vi "LoadZstackImages.vi"(0 "Experiment folder path OR Z-stack folder path":path, 11 "Error In":errorcluster) -> (1 "Number of Files":i32, 2 "All outputs":T2, 3 "AOL Z Planes":dbl[](array[numeric]), 4 "RedImageArray":T1[](array[typedef]), 6 "GreenImageArray":T1[](array[typedef]), 8 "Motor Z planes":dbl[](array[numeric]), 10 "AOL Z Planes (norm)":dbl[](array[numeric]), 12 "RedMaxZ":T1, 14 "GreenMaxZ":T1, 15 "Error Out":errorcluster)   [LabVIEW 2013]
uses:
  <vilib>/vision/Image Controls.llb/IMAQ Image.ctl
  <vilib>/vision/NI_Vision_Development_Module.lvlib
panel:
  out "Green":path[](array[path])
  out "Red":path[](array[path])
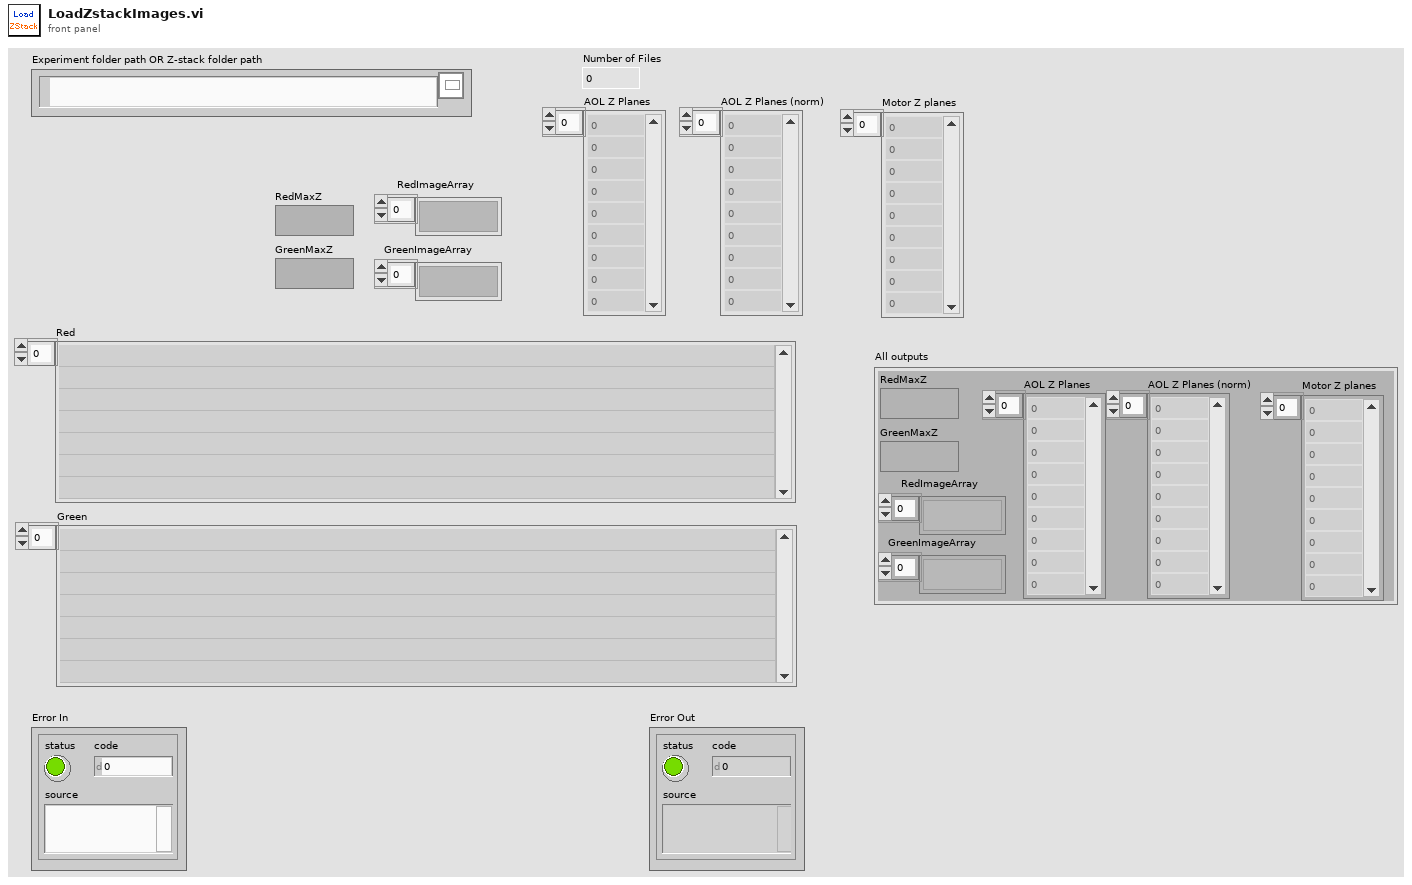
[diagram p1: front panel]
types:
  T1 = typedef "IMAQ Image.ctl" = refnum<image>
  T2 = cluster{"RedImageArray":T1[], "GreenImageArray":T1[], "RedMaxZ":T1, "GreenMaxZ":T1, "AOL Z Planes":dbl[], "AOL Z Planes (norm)":dbl[], "Motor Z planes":dbl[]}
  T3 = typedef "Fixed strings.ctl" = cluster{"ROI file name":string, "Normalised ROI file name":string, "Zplane Pockels values file name":string, "Functional data folder name":string, "Experiment Header file name":string, "Z-stack images folder name":string, "Groups setup rel. path":string, "Groups text file rel. path":string, "TDMS files folder name (F.img)":string, "TDMS files folder name (V.acq)":string, "TDMS files folder name (Pl.acq)":string, "Cycle rel times sequence file":string, "Dynamically called VIs folder name":string, "Time Series folder base name":string}
  T4 = enum32{"Average", "Min", "Max", "Clear  if < ", "Clear  if < or =", "Clear  if =", "Clear  if > or =", "Clear  if >"}
  T5 = typedef "Image Type" = u32
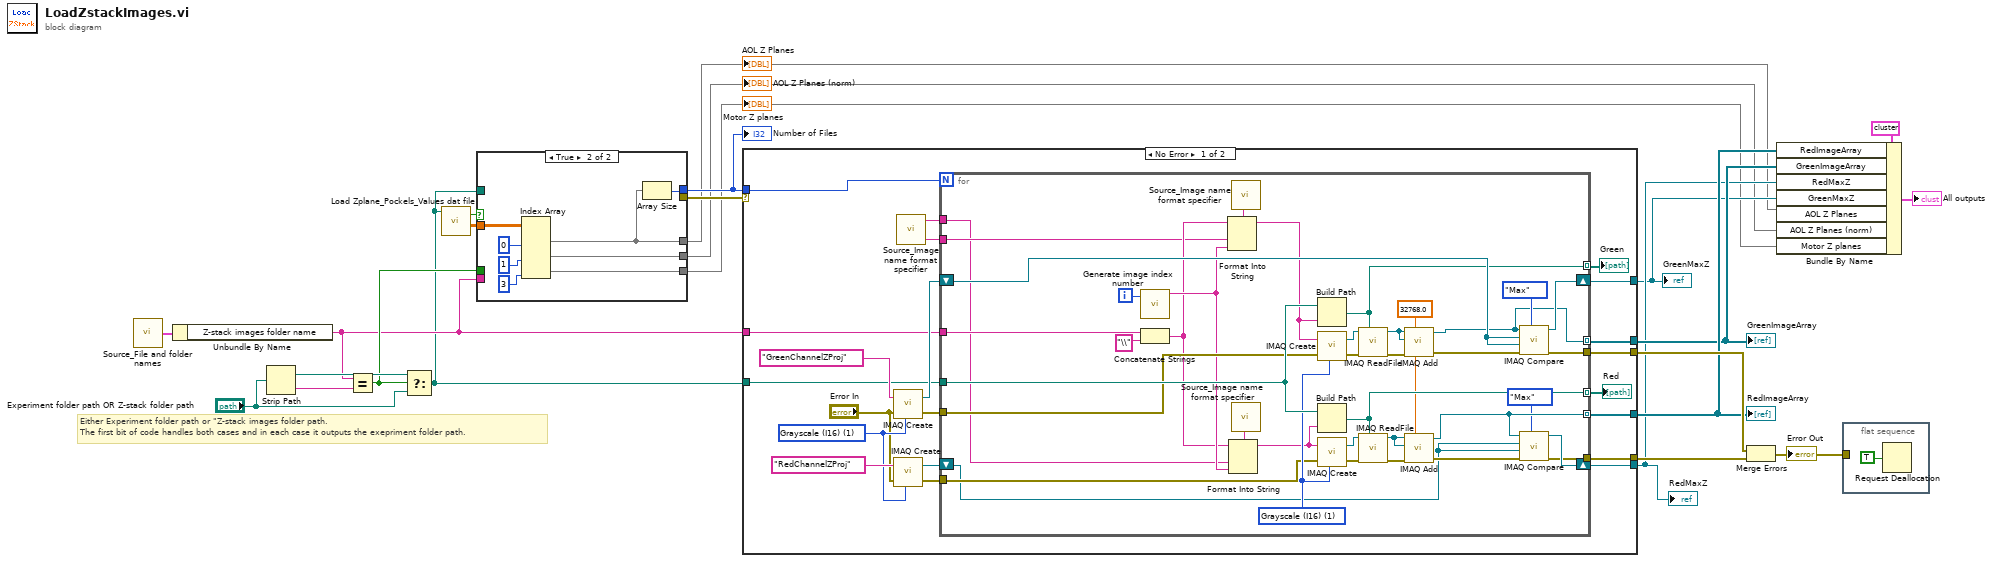
[diagram p0: block diagram]
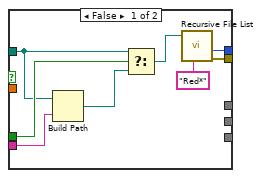
[diagram p2: hidden frame]
diagram:
  # "Either Experiment folder path or \"Z-stack images folder path.\nThe first bit of code handles both cases and in each case it outputs the exepriment folder path."
  n1 = call "Source_File and folder names.vi"() -> ("Fixed strings"=w15:T3)  [unwired: 1 in]
  n2 = Unbundle By Name(w15) -> ("Z-stack images folder name"=w14:string)
  n3 = Strip Path(path="Experiment folder path OR Z-stack folder path") -> (stripped path=w21:path, name=w18:string)
  n4 = Equal?(x=w14, y=w18) -> (x = y?=w20:bool)
  n5 = Select(t=w21, s=w20, f="Experiment folder path OR Z-stack folder path") -> (s? t:f=w1:path)
  n6 = call "Load Zplane_Pockels_Values dat file.vi"("Experiment data folder path"=w1) -> ("Zplane_Pockels_Values file data (header removed)"=w13:dbl[][], "Zplane Pockels values file exists"=w12:bool)  [unwired: 5 in, 4 out]
  n7 = case shown="True" w12 {
    tunnel: [w30 w38] -> w16
    tunnel: w1 -> [w27 _]
    tunnel: w14 -> [w29 _]
    tunnel: w20 -> [w28 _]
    tunnel: [w24 _] -> w19
    tunnel: [_ w36] -> w4
    tunnel: [_ w35] -> w3
    tunnel: w13 -> [_ w34]
    tunnel: [_ w32] -> w2
    frame False {
      n8 = Build Path(base path=w27, name or relative path=w29) -> (appended path=w26:path)
      n9 = Select(t=w27, s=w28, f=w26) -> (s? t:f=w25:path)
      n10 = call <vilib>:"Recursive File List.vi"("pattern"="Red*", "Folder Path"=w25) -> ("error out"=w24:errorcluster, "Number of Files"=w30:i32)  [unwired: 5 in, 3 out]
    }
    frame True {
      n11 = Index Array(array=w34, index (col) #1=0 ("disabled index (col)"), index (col) #2=1 ("disabled index (row)"), index (col) #3=3 ("index (col)")) -> (element #1=w36:dbl[], element #2=w35:dbl[], element #3=w32:dbl[])  [unwired: 3 in]
      n12 = Array Size(array=w36) -> (size(s)=w38:i32)
    }
  }
  "AOL Z Planes" <- w4
  "AOL Z Planes (norm)" <- w3
  "Number of Files" <- w16
  "Motor Z planes" <- w2
  n13 = case shown="No Error" w19 {
    selector: w19 -> [_ w99]
    tunnel: [w60 _] -> w7
    tunnel: [w59 _] -> w5
    tunnel: [w50 _] -> w8
    tunnel: [w49 _] -> w23
    tunnel: [w48 w99] -> w22
    tunnel: [w47 _] -> w6
    tunnel: w16 -> [w46 _]
    tunnel: w14 -> [w45 _]
    tunnel: w1 -> [w44 _]
    frame No Error {
      w52 = T5 1 items=["Grayscale (U8)", "Grayscale (I16)", "Grayscale (SGL)", "Complex (CSG)", "RGB (U32)", "HSL (U32)", "RGB (U64)"] ("Image Type")
      n14 = call "IMAQ Create"("Image Name"="GreenChannelZProj" ("string"), "Image Type"=w52, "error in (no error)"="Error In") -> ("New Image"=w55:T1, "error out"=w56:errorcluster)  [unwired: 2 in]
      n15 = call "IMAQ Create"("Image Name"="RedChannelZProj" ("string"), "Image Type"=w52, "error in (no error)"="Error In") -> ("New Image"=w57:T1, "error out"=w58:errorcluster)  [unwired: 2 in]
      n16 = call "Source_Image name format specifier.vi"() -> ("Red channel name"=w41:string, "Green channel name"=w40:string)  [unwired: 5 in, 1 out]
      n17 = for {
        N: w46 -> [_]
        tunnel: [w78] -> w50 mode=indexing
        tunnel: [w61] -> w60 mode=indexing
        tunnel: w44 -> [w94]
        shift-right: [w62] -> w59
        shift-left: w55 -> [w89]
        tunnel: [w93] -> w48
        tunnel: w56 -> [w83]
        shift-right: [w92] -> w47
        shift-left: w57 -> [w74]
        tunnel: w58 -> [w82]
        tunnel: [w91] -> w49
        tunnel: w45 -> [w76]
        tunnel: [w69] -> w43 mode=indexing
        tunnel: [w66] -> w42 mode=indexing
        tunnel: w40 -> [w65]
        tunnel: w41 -> [w64]
        i -> [w87]
        w63 = 32768.0 ("Constant")
        w88 = T5 1 items=["Grayscale (U8)", "Grayscale (I16)", "Grayscale (SGL)", "Complex (CSG)", "RGB (U32)", "HSL (U32)", "RGB (U64)"] ("Image Type")
        n18 = call "Generate image index number.vi"("FOR loop iteration or existing number of files"=w87) -> ("Number in string representation (padded with zeroes)"=w72:string)  [unwired: 10 in]
        n19 = Concatenate Strings(w76, "\\" ("string")) -> (w70:string)
        n20 = call "Source_Image name format specifier.vi"() -> ("Z-Stack Image name format specifier"=w68:string)  [unwired: 5 in, 2 out]
        n21 = Format Into String(format string=w68, initial string=w70, w65, w72) -> (resulting string=w73:string)  [unwired: 1 in, 1 out]
        n22 = call "Source_Image name format specifier.vi"() -> ("Z-Stack Image name format specifier"=w67:string)  [unwired: 5 in, 2 out]
        n23 = Format Into String(format string=w67, initial string=w70, w64, w72) -> (resulting string=w71:string)  [unwired: 1 in, 1 out]
        n24 = Build Path(base path=w94, name or relative path=w73) -> (appended path=w66:path)
        n25 = call "IMAQ Create"("Image Name"=w73, "Image Type"=w88, "error in (no error)"=w83) -> ("New Image"=w96:T1, "error out"=w95:errorcluster)  [unwired: 2 in]
        n26 = Build Path(base path=w94, name or relative path=w71) -> (appended path=w69:path)
        n27 = call "IMAQ Create"("Image Name"=w71, "Image Type"=w88, "error in (no error)"=w82) -> ("New Image"=w97:T1, "error out"=w98:errorcluster)  [unwired: 2 in]
        n28 = call "IMAQ ReadFile"("File Path"=w66, "error in (no error)"=w95, "Image"=w96) -> ("error out"=w84:errorcluster, "Image Out"=w86:T1)  [unwired: 4 in, 3 out]
        n29 = call "IMAQ ReadFile"("File Path"=w69, "error in (no error)"=w98, "Image"=w97) -> ("error out"=w81:errorcluster, "Image Out"=w85:T1)  [unwired: 4 in, 3 out]
        n30 = call "IMAQ Add"("Image Src A"=w86, "Constant"=w63, "Image Dst"=w86, "error in (no error)"=w84) -> ("Image Dst Out"=w61:T1, "error out"=w79:errorcluster)  [unwired: 3 in]
        n31 = call "IMAQ Add"("Image Src A"=w85, "Constant"=w63, "Image Dst"=w85, "error in (no error)"=w81) -> ("Image Dst Out"=w78:T1, "error out"=w80:errorcluster)  [unwired: 3 in]
        n32 = call "IMAQ Compare"("Operator"=T4."Max", "error in (no error)"=w79, "Image Src B"=w89, "Image Dst"=w89, "Image Src A"=w61) -> ("error out"=w93:errorcluster, "Image Dst Out"=w62:T1)  [unwired: 5 in]
        n33 = call "IMAQ Compare"("Operator"=T4."Max", "error in (no error)"=w80, "Image Src B"=w74, "Image Dst"=w74, "Image Src A"=w78) -> ("error out"=w91:errorcluster, "Image Dst Out"=w92:T1)  [unwired: 5 in]
      }
      "Red" <- w43
      "Green" <- w42
    }
    frame Error {
    }
  }
  "RedImageArray" <- w8
  "GreenImageArray" <- w7
  "RedMaxZ" <- w6
  "GreenMaxZ" <- w5
  n34 = Merge Errors(w22, w23) -> (w11:errorcluster)
  "Error Out" <- w11
  n35 = Bundle By Name(cluster=T2 {"RedImageArray"=[], "GreenImageArray"=[], "RedMaxZ"=refnum, "GreenMaxZ"=refnum, "AOL Z Planes"=[], "AOL Z Planes (norm)"=[], "Motor Z planes"=[]} ("All outputs"), "RedImageArray"=w8, "GreenImageArray"=w7, "RedMaxZ"=w6, "GreenMaxZ"=w5, "AOL Z Planes"=w4, "AOL Z Planes (norm)"=w3, "Motor Z planes"=w2) -> (→"All outputs":T2)
  n36 = flat-sequence {
    tunnel: w11 -> [_]
    frame #0 {
      n37 = Request Deallocation(TRUE ("flag")) -> ()
    }
  }
